vi "PickPlace_org.vi"(4 "Tool or Plate":enum16{"Tool", "Plate"}(ring), 5 "Pick or Drop":enum16{"Pick", "Drop"}(ring)) -> (0 "error out":errorcluster, 2 "sensor on?":bool)   [LabVIEW 2019]
uses:
  Other Models/2010/Motion/AbortSingle.vi
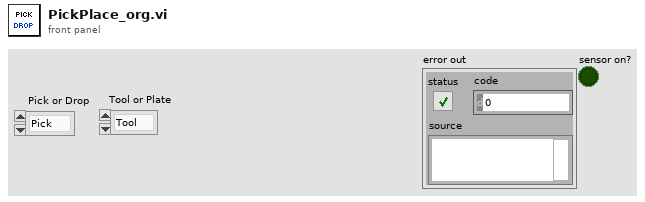
[diagram p1: front panel]
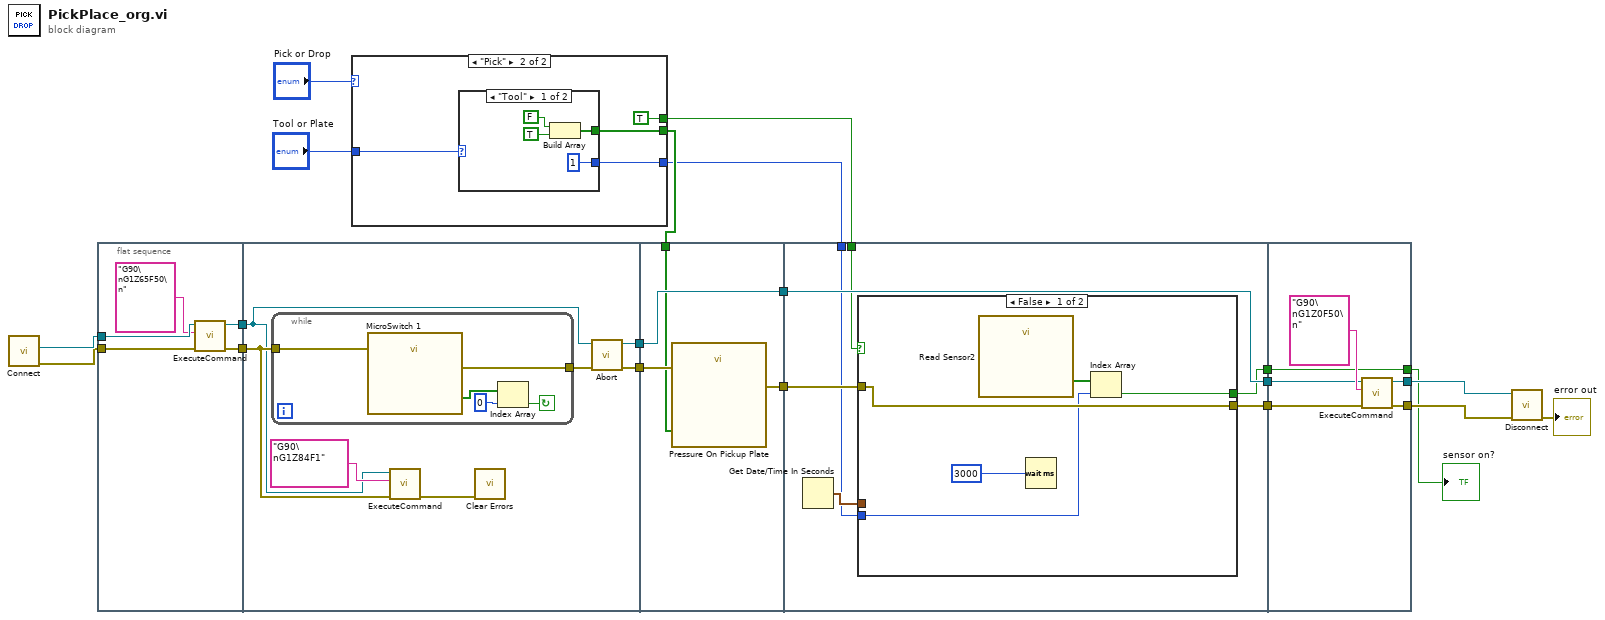
[diagram p0: block diagram]
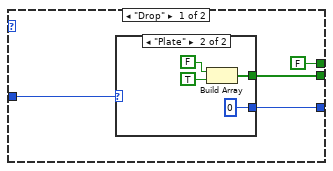
[diagram p2: hidden frame]
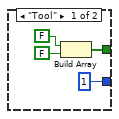
[diagram p3: hidden frame]
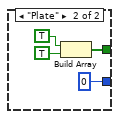
[diagram p4: hidden frame]
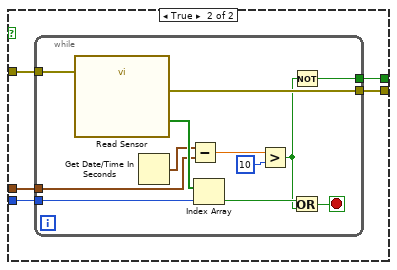
[diagram p5: hidden frame]
diagram:
  n1 = call "Connect.vi"() -> ("error out"=w19:errorcluster, "controller"=w20:refnum<k24>)  [unwired: 10 in]
  n2 = flat-sequence {
    tunnel: w20 -> [w25]
    tunnel: w19 -> [w23]
    tunnel: [w24] -> w18
    tunnel: [w22] -> w17
    tunnel: w18 -> [w28]
    tunnel: w17 -> [w31]
    tunnel: [w29] -> w16
    tunnel: [w27] -> w15
    tunnel: w16 -> [w41]
    tunnel: w15 -> [w40]
    tunnel: [w41] -> w14
    tunnel: [w39] -> w13
    tunnel: w5 -> [w38]
    tunnel: w14 -> [w48]
    tunnel: w13 -> [w47]
    tunnel: [w48] -> w12
    tunnel: [w45] -> w11
    tunnel: [w44] -> w7
    tunnel: w4 -> [w43]
    tunnel: w3 -> [w42]
    tunnel: w12 -> [w74]
    tunnel: w11 -> [w75]
    tunnel: [w73] -> w10
    tunnel: [w72] -> w9
    tunnel: [w71] -> w8
    tunnel: w7 -> [w71]
    frame #0 {
      n3 = call "ExecuteCommand.vi"("error in (no error)"=w23, "Command Code"="G90\nG1Z65F50\n", "controller in"=w25) -> ("error out"=w22:errorcluster, "controller out"=w24:refnum<k24>)  [unwired: 6 in, 1 out]
    }
    frame #1 {
      n4 = while {
        tunnel: [w37] -> w30
        tunnel: w31 -> [w36]
        stop <- w34 continue-if-true
        n5 = call "MicroSwitch 1"("error in"=w36) -> ("data"=w35:bool[], "error out"=w37:errorcluster)  [unwired: 16 in, 1 out]
        n6 = Index Array(array=w35, index=0) -> (element=w34:bool)
      }
      n7 = call "ExecuteCommand.vi"("error in (no error)"=w31, "Command Code"="G90\nG1Z84F1", "controller in"=w28) -> ("error out"=w26:errorcluster)  [unwired: 6 in, 2 out]
      n8 = call <vilib>:"Clear Errors.vi"("error in (no error)"=w26) -> ()  [unwired: 5 in, 2 out]
      n9 = call-poly "Abort.vi"("error in (no error)"=w30, "controller in"=w28) -> ("error out"=w27:errorcluster, "controller out"=w29:refnum<k24>)  [unwired: 8 in]
    }
    frame #2 {
      n10 = call "Pressure On Pickup Plate"("data"=w38, "error in"=w40) -> ("error out"=w39:errorcluster)  [unwired: 16 in, 1 out]
    }
    frame #3 {
      n11 = Get Date/Time In Seconds() -> (seconds since 1Jan1904=w46:timestamp)
      n12 = case shown="False" w42 {
        tunnel: w47 -> [w53 w58]
        tunnel: w46 -> [_ w57]
        tunnel: [w53 w56] -> w45
        tunnel: [w50 w55] -> w44
        tunnel: w43 -> [w51 w54]
        frame False {
          n13 = call "Read Sensor2"() -> ("data"=w52:bool[])  [unwired: 17 in, 2 out]
          n14 = Wait (ms)(milliseconds to wait=3000) -> ()  [unwired: 1 out]
          n15 = Index Array(array=w52, index=w51) -> (element=w50:bool)
        }
        frame True {
          n16 = while {
            tunnel: w58 -> [w69]
            tunnel: w57 -> [w65]
            tunnel: [w63] -> w56
            tunnel: [w62] -> w55
            tunnel: w54 -> [w61]
            stop <- w64 stop-if-true
            n17 = call "Read Sensor"("error in"=w69) -> ("data"=w70:bool[], "error out"=w63:errorcluster)  [unwired: 16 in, 1 out]
            n18 = Get Date/Time In Seconds() -> (seconds since 1Jan1904=w68:timestamp)
            n19 = Subtract(x=w68, y=w65) -> (x-y=w66:dbl)
            n20 = Index Array(array=w70, index=w61) -> (element=w60:bool)
            n21 = Greater?(x=w66, y=10) -> (0:w59:bool)
            n22 = Not(x=w59) -> (.not. x?=w62:bool)
            n23 = Or(x=w60, y=w59) -> (x .or. y?=w64:bool)
          }
        }
      }
    }
    frame #4 {
      n24 = call "ExecuteCommand.vi"("error in (no error)"=w75, "Command Code"="G90\nG1Z0F50\n", "controller in"=w74) -> ("error out"=w72:errorcluster, "controller out"=w73:refnum<k24>)  [unwired: 6 in, 1 out]
    }
  }
  n25 = case shown="\"Pick\"" "Pick or Drop" {
    tunnel: "Tool or Plate" -> [w77 w92]
    tunnel: [w80 w91] -> w5
    tunnel: [w79 w90] -> w4
    tunnel: [FALSE TRUE] -> w3
    frame "Drop" {
      n26 = case shown="\"Plate\"" w77 {
        tunnel: [w82 w86] -> w80
        tunnel: [1 0] -> w79
        frame "Tool" {
          n27 = Build Array(FALSE, FALSE) -> (w82:bool[])
        }
        frame "Plate" {
          n28 = Build Array(FALSE, TRUE) -> (w86:bool[])
        }
      }
    }
    frame "Pick" {
      n29 = case shown="\"Tool\"" w92 {
        tunnel: [w94 w98] -> w91
        tunnel: [1 0] -> w90
        frame "Tool" {
          n30 = Build Array(FALSE, TRUE) -> (w94:bool[])
        }
        frame "Plate" {
          n31 = Build Array(TRUE, TRUE) -> (w98:bool[])
        }
      }
    }
  }
  n32 = call "Disconnect.vi"("error in (no error)"=w9, "controller"=w10) -> ("error out"=→"error out":errorcluster)  [unwired: 9 in]
  "sensor on?" <- w8
